vi "Diag_SnapInfo.vi"(0 "GEA2 Reference In":refnum<k24>, 5 "GEA Inputs":T2 {"Destination" format="%.0x"; "Source" format="%.0x"}, 7 "Table Entry Count":u16, 9 "Table Status Location":u16 format="%.0x", 11 "Error In":errorcluster) -> (4 "GEA2 Reference Out":refnum<k24>, 6 "Snap Location":T1[](array[typedef]) {"ERD Number" format="%.0x"}, 8 "Raw Snap Data":string[](array[string]), 15 "Error Out":errorcluster)   [LabVIEW 2023]
uses:
  LabVIEW GEA2 Toolkit/GEA3/type defs/Source_Destination.ctl
  D:/Common/LabVIEW GEA2 Toolkit/source/GEA3 DLL Source/GeaCommunication.dll
  LabVIEW GEA2 Toolkit/source/GEA3 DLL Source/GeaCommunication.dll
  LabVIEW GEA2 Toolkit/GEA3/type defs/ERD Read Data In.ctl
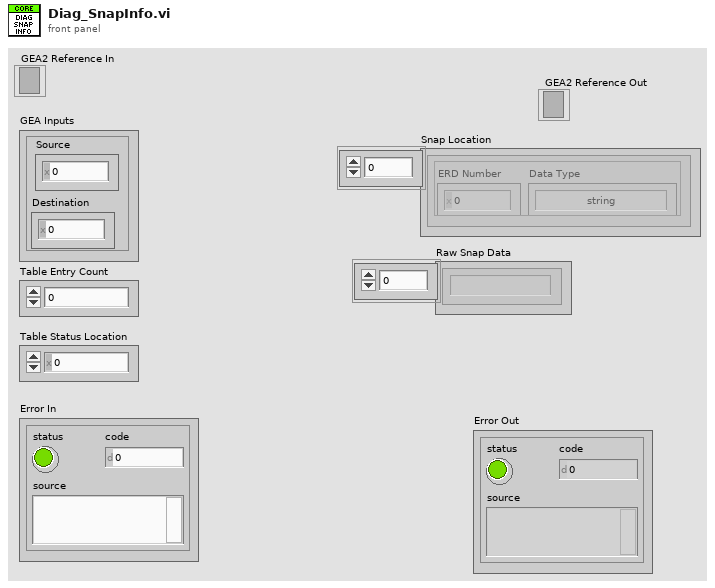
[diagram p1: front panel]
types:
  T1 = typedef "ERD Read Data In.ctl" = cluster{"ERD Number":u16, "Data Type":enum16{"string", "boolean", "uint8_t", "uint16_t", "uint32_t", "uint64_t", "int8_t", "int16_t", "int32_t", "int64_t"}}
  T2 = typedef "Source_Destination.ctl" = cluster{"Source":u8, "Destination":u8}
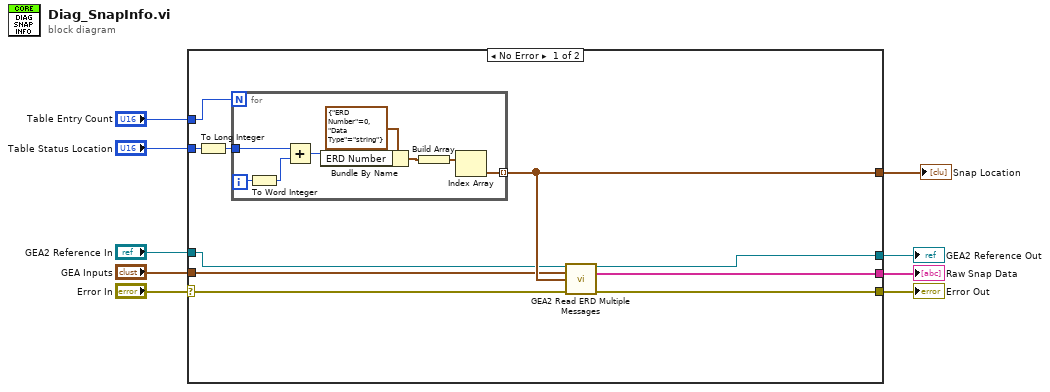
[diagram p0: block diagram]
diagram:
  n1 = case shown="No Error" "Error In" {
    selector: "Error In" -> [w15 w28]
    tunnel: [w14 w28] -> w4
    tunnel: "Table Status Location" -> [w11 _]
    tunnel: "Table Entry Count" -> [w19 _]
    tunnel: "GEA Inputs" -> [w17 _]
    tunnel: "GEA2 Reference In" -> [w16 _]
    tunnel: [w18 _] -> w3
    tunnel: [w13 _] -> w1
    tunnel: [w12 _] -> w2
    frame No Error {
      n2 = To Long Integer(number=w11) -> (32bit integer=w10:i32)
      n3 = for {
        N: w19 -> [_]
        tunnel: w10 -> [w27]
        tunnel: [w22] -> w18 mode=indexing
        i -> [w21]
        n4 = To Word Integer(number=w21) -> (16bit integer=w20:i16)
        n5 = Add(x=w27, y=w20) -> (x+y=w26:i32)
        n6 = Bundle By Name(cluster=T1 {"ERD Number"=0, "Data Type"=enum."string"} ("ERD Read Data In"), "ERD Number"=w26) -> (w24:T1)
        n7 = Build Array(w24) -> (w23:T1[])
        n8 = Index Array(array=w23) -> (element=w22:T1)  [unwired: 1 in]
      }
      n9 = call "GEA2 Read ERD Multiple Messages.vi"("GEA2 Reference In"=w16, "GEA Inputs"=w17, "Read ERD List"=w18, "Error In"=w15) -> ("GEA2 Reference Out"=w12:refnum<k24>, "Raw Data Out"=w13:string[], "Error Out"=w14:errorcluster)  [unwired: 8 in, 1 out]
    }
    frame Error {
    }
  }
  "Error Out" <- w4
  "Snap Location" <- w3
  "GEA2 Reference Out" <- w2
  "Raw Snap Data" <- w1
